vi "fileIO.vi"   [LabVIEW 2015]
types:
  T1 = enum16{"open", "replace", "create", "open or create", "replace or create", "replace or create with confirmation"}
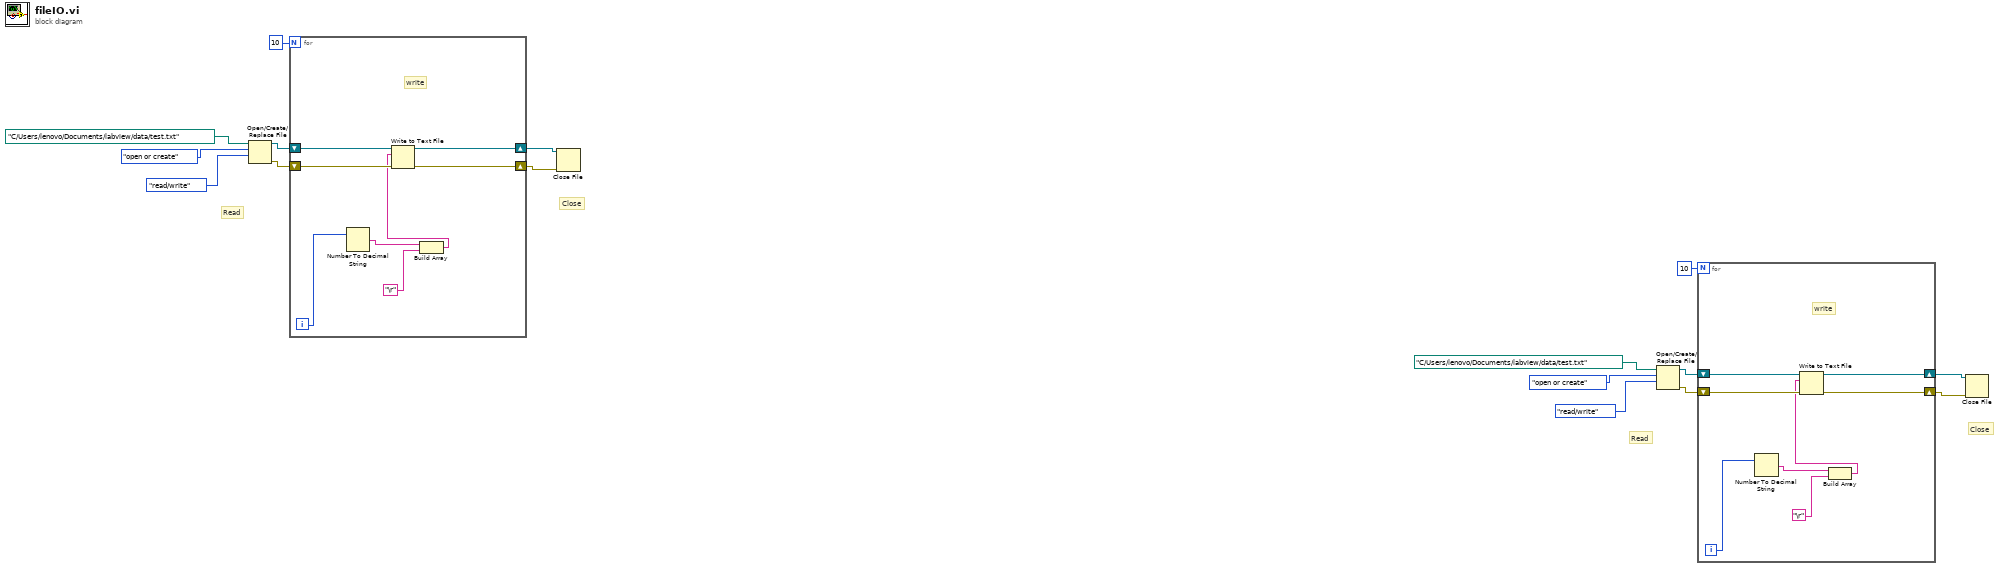
[diagram p0: block diagram]
diagram:
  # "Read"
  # "Close"
  # "Read"
  # "Close"
  n1 = Open/Create/Replace File(file path (use dialog)=path "C:/Users/lenovo/Documents/labview/data/test.txt", operation (0:open)=T1."open or create", access (0:read/write)=enum16{"read/write", "read-only", "write-only"}."read/write") -> (refnum out=w4:refnum<file>, error out=w3:errorcluster)  [unwired: 3 in, 1 out]
  n2 = for {
    N: 10 -> [_]
    shift-right: [w21] -> w1
    shift-left: w4 -> [w24]
    shift-right: [w22] -> w2
    shift-left: w3 -> [w23]
    i -> [w20]
    # "write"
    n3 = Number To Decimal String(number=w20) -> (decimal integer string=w19:string)  [unwired: 1 in]
    n4 = Build Array(w19, "\r") -> (w17:string[])
    n5 = Write to Text File(file (use dialog)=w24, text=w17, error in=w23) -> (refnum out=w21:refnum<file>, error out=w22:errorcluster)  [unwired: 1 in, 1 out]
  }
  n6 = Close File(refnum=w1, error in=w2) -> ()  [unwired: 2 out]
  n7 = Open/Create/Replace File(file path (use dialog)=path "C:/Users/lenovo/Documents/labview/data/test.txt", operation (0:open)=T1."open or create", access (0:read/write)=enum16{"read/write", "read-only", "write-only"}."read/write") -> (refnum out=w12:refnum<file>, error out=w11:errorcluster)  [unwired: 3 in, 1 out]
  n8 = for {
    N: 10 -> [_]
    shift-right: [w29] -> w9
    shift-left: w12 -> [w32]
    shift-right: [w30] -> w10
    shift-left: w11 -> [w31]
    i -> [w28]
    # "write"
    n9 = Number To Decimal String(number=w28) -> (decimal integer string=w27:string)  [unwired: 1 in]
    n10 = Build Array(w27, "\r") -> (w25:string[])
    n11 = Write to Text File(file (use dialog)=w32, text=w25, error in=w31) -> (refnum out=w29:refnum<file>, error out=w30:errorcluster)  [unwired: 1 in, 1 out]
  }
  n12 = Close File(refnum=w9, error in=w10) -> ()  [unwired: 2 out]
